vi "HDF5_append-dataset-2D.vi"() -> ()   [LabVIEW 2018]
uses:
  <vilib>/addons/h5labview2/file/H5Fmode.ctl
  HDF5/HDF5_ToneInfoClust.ctl
  <vilib>/addons/h5labview2/file/H5F.lvlib
  <vilib>/addons/h5labview2/dataset/H5D.lvlib
panel:
  in  "data":i32[][](array[numeric])=[[0, 1, 2, 3, 4], [5, 6, 7, 8, 9]]
  out "ms/append":dbl
  out "timer (ms)":u32
  out "progress":i32(slide)=9999 scale=0.0..10.0
  in  "repetitions":i32=1000
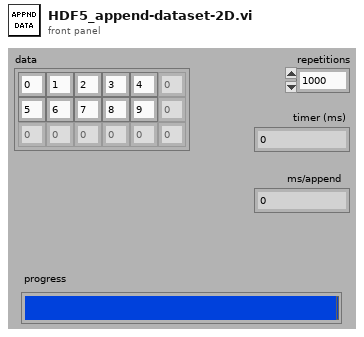
[diagram p1: front panel]
types:
  T1 = typedef "H5F.lvlib/H5Fmode.ctl" = enum16{"read-only", "read-write", "overwrite", "create new", "open or create"}
  T2 = typedef "HDF5_ToneInfoClust.ctl" = cluster{"Timestring":string, "Timestamp":dbl, "MaxValue":dbl, "PeakLoc":dbl, "df":dbl}
  T3 = typedef "hid_t.ctl" = i32
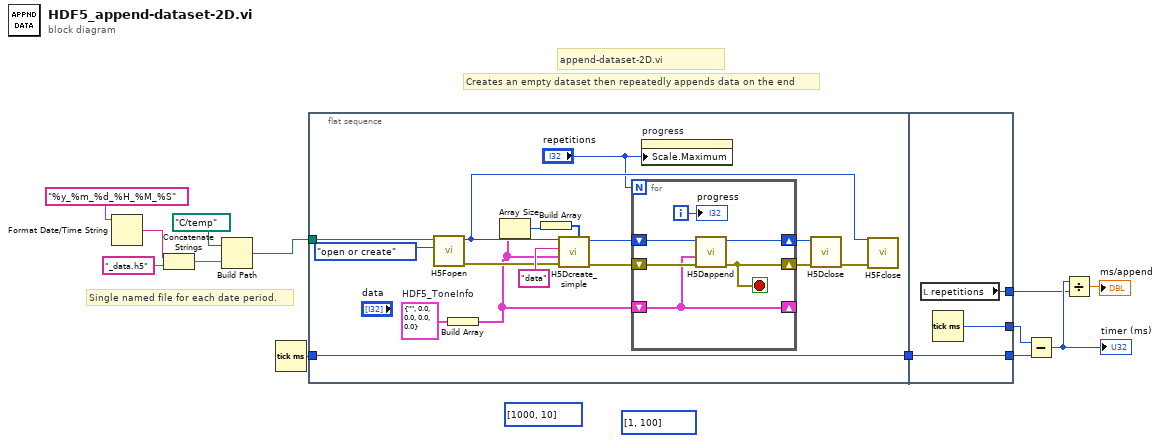
[diagram p0: block diagram]
diagram:
  (unwired) u64[] [1, 100] ("chunk size")
  (unwired) u64[] [1000, 10] ("max size")
  # "Single named file for each date period."
  # "Creates an empty dataset then repeatedly appends data on the end"
  # "append-dataset-2D.vi"
  n1 = Format Date/Time String(time format string (%c)="%y_%m_%d_%H_%M_%S") -> (date/time string=w3:string)  [unwired: 2 in]
  n2 = Concatenate Strings(w3, "_data.h5" ("string")) -> (w5:string)
  n3 = Build Path(base path=path "C:/temp", name or relative path=w5) -> (appended path=w1:path)
  n4 = Tick Count (ms)() -> (millisecond timer value=w13:u32)
  n5 = flat-sequence {
    tunnel: w13 -> [w23]
    tunnel: [w23] -> w12
    tunnel: w1 -> [w18]
    tunnel: w12 -> [w37]
    tunnel: [w38] -> w11
    tunnel: [w37] -> w10
    tunnel: [w36] -> w8
    frame #0 {
      w17 = T2 {"Timestring"="", "Timestamp"=0.0, "MaxValue"=0.0, "PeakLoc"=0.0, "df"=0.0}  # HDF5_ToneInfo
      n6 = call <vilib>:"H5Fopen.vi"("mode (read-only)"=H5Fmode."open or create" ("mode"), "path"=w18) -> ("error out"=w25:errorcluster, "ref out"=w24:T3)  [unwired: 8 in]
      n7 = Build Array(w17) -> (w16:T2[])
      n8 = Array Size(array=w16) -> (size(s)=w15:i32)
      n9 = Build Array(w15) -> (w14:i32[])
      n10 = call <vilib>:"H5Dcreate_simple.vi"("chunk size"=w14, "error in (no error)"=w25, "type in"=w16, "name"="data", "ref in"=w24) -> ("error out"=w26:errorcluster, "dset out"=w27:T3)  [unwired: 5 in]
      n11 = for {
        N: "repetitions" -> [_]
        shift-right: [w33] -> w21
        shift-left: w26 -> [w34]
        shift-right: [w30] -> _
        shift-left: w16 -> [w30]
        shift-right: [w32] -> w20
        shift-left: w27 -> [w31]
        i -> [w35]
        stop <- w33 stop-if-true
        n12 = call <vilib>:"H5Dappend.vi"("error in (no error)"=w34, "data"=w30, "ref in"=w31) -> ("error out"=w33:errorcluster, "ref out"=w32:T3)  [unwired: 5 in, 2 out]
        "progress" <- w35
      }
      n13 = property on="progress" class="Slide (strict)"("Scale.Maximum"="repetitions") -> ()  [unwired: 2 in, 2 out]
      n14 = call <vilib>:"H5Dclose.vi"("error in (no error)"=w21, "dset in"=w20) -> ("error out"=w19:errorcluster)  [unwired: 9 in]
      n15 = call <vilib>:"H5Fclose.vi"("error in (no error)"=w19, "ref"=w24) -> ()  [unwired: 9 in, 1 out]
    }
    frame #1 {
      n16 = local read "repetitions"() -> (w36:i32)
      n17 = Tick Count (ms)() -> (millisecond timer value=w38:u32)
    }
  }
  n18 = Subtract(x=w11, y=w10) -> (x-y=w9:u32)
  "timer (ms)" <- w9
  n19 = Divide(x=w9, y=w8) -> (x/y=→"ms/append":dbl)
